vi "FTDI - Byte to Float.vi"(11 "Byte":u8[](array[numeric])) -> (3 "Float":sgl)   [LabVIEW 2019]
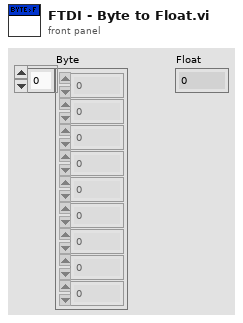
[diagram p1: front panel]
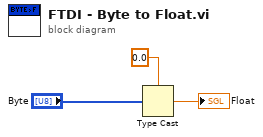
[diagram p0: block diagram]
diagram:
  n1 = Type Cast(type=sgl 0.0 ("Float"), x="Byte") -> (*(type *) &x=→"Float":sgl)
